vi "Temp F to C.vi"() -> ()   [LabVIEW 2020]
panel:
  in  "stop":bool
  out "Temp(C)":dbl
  out "Waveform Chart":dbl(graph)
  in  "Thermometer":dbl(slide) scale=0.0..100.0
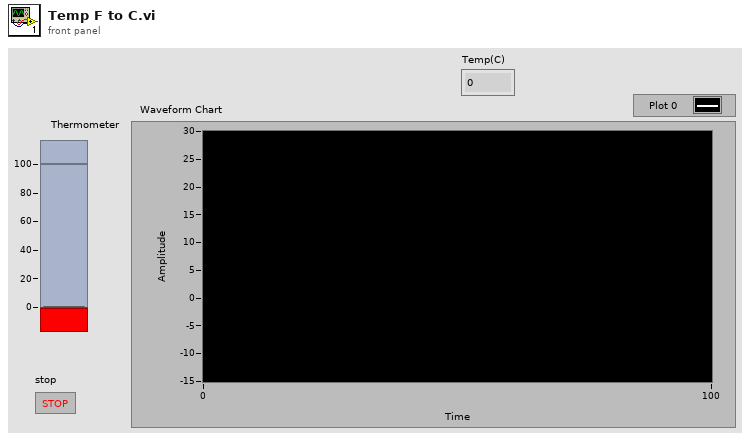
[diagram p1: front panel]
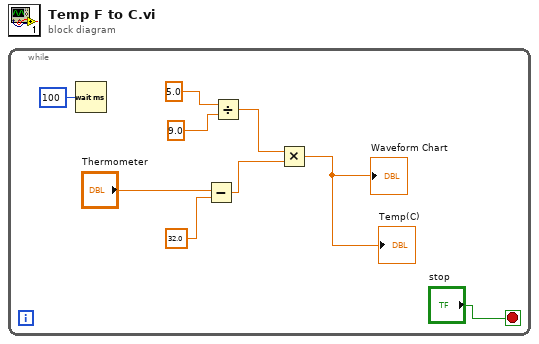
[diagram p0: block diagram]
diagram:
  n1 = while {
    stop <- "stop" stop-if-true
    n2 = Wait (ms)(milliseconds to wait=u32 100) -> ()  [unwired: 1 out]
    n3 = Subtract(x="Thermometer", y=32.0) -> (x-y=w4:dbl)
    n4 = Divide(x=5.0, y=9.0) -> (x/y=w3:dbl)
    n5 = Multiply(x=w3, y=w4) -> (x*y=→"Waveform Chart" →"Temp(C)":dbl)
  }
